vi "试剂余量展示.vi"(11 "波形图 2":refnum<vi>) -> (3 "波形图":sgl[][](graph))   [LabVIEW 2016, in "斯坦道氟化物.lvlib"]
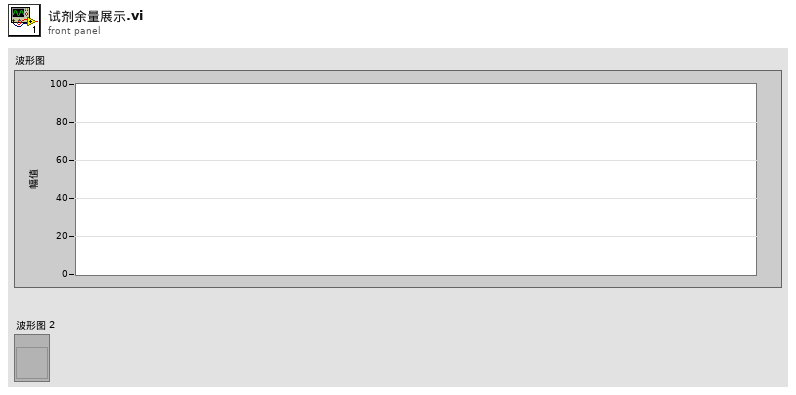
[diagram p1: front panel]
types:
  T1 = cluster{"Name":string, "Color":u32, "Style":u8, "Point Style":u8, "Name Visible":bool, "Allow Drag":bool, "Annotation Mode":u32, "Plot":i32, "Index":i32, "Position":cluster{"X":dbl, "Y":i32}, "X Scale":u32, "Y Scale":u32, "Show Arrow":bool, "Lock Name":bool, "Plot Area":i32, "Label Offset":cluster{"X":dbl, "Y":dbl}}[]
  T2 = cluster{"V1":sgl, "V2":sgl, "V3":sgl, "V4":sgl, "V5":sgl, "V6":sgl, "V7":sgl, "V8":sgl, "V9":sgl, "V10":sgl, "V11":sgl, "V12":sgl, "V9-1":sgl, "V9-2":sgl}
  T3 = cluster{"V":string, "V 2":string, "V 3":string, "V 4":string, "V 5":string, "V 6":string, "V 7":string, "V 8":string, "V 9":string, "V 10":string, "V 11":string, "V 12":string, "V9-1":string, "V9-2":string}
  T4 = cluster{"Name":string, "Color":u32, "Style":u8, "Point Style":u8, "Name Visible":bool, "Allow Drag":bool, "Annotation Mode":u32, "Plot":i32, "Index":i32, "Position":cluster{"X":dbl, "Y":i32}, "X Scale":u32, "Y Scale":u32, "Show Arrow":bool, "Lock Name":bool, "Plot Area":i32, "Label Offset":cluster{"X":dbl, "Y":dbl}}
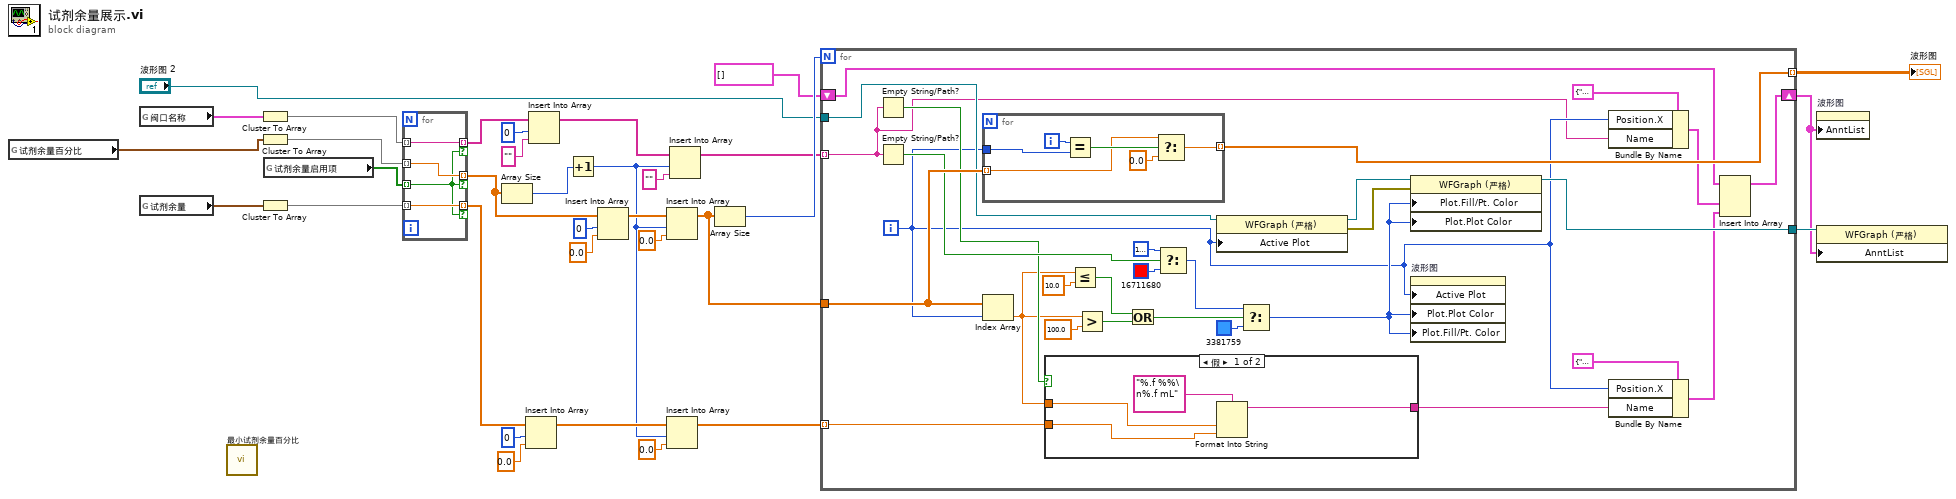
[diagram p0: block diagram]
diagram:
  n1 = global read "VAR总磷总氮全局变量.vi" "试剂余量百分比"() -> (w33:T2)
  n2 = global read "总磷总氮断电保存全局变量.vi" "阀口名称"() -> (w22:T3)
  n3 = global read "VAR总磷总氮全局变量.vi" "试剂余量"() -> (w11:T2)
  n4 = call "最小试剂余量百分比.vi"() -> ()  [unwired: 12 in]
  n5 = Cluster To Array(cluster=w22) -> (array=w21:string[])
  n6 = Cluster To Array(cluster=w33) -> (array=w32:sgl[])
  n7 = Cluster To Array(cluster=w11) -> (array=w10:sgl[])
  n8 = global read "VAR总磷总氮全局变量.vi" "试剂余量启用项"() -> (w31:bool[])
  n9 = for {
    tunnel: w32 -> [w37] mode=indexing
    tunnel: w31 -> [w34] mode=indexing
    tunnel: [w37] -> w30 mode=indexing if=w34
    tunnel: w21 -> [w36] mode=indexing
    tunnel: [w36] -> w20 mode=indexing if=w34
    tunnel: w10 -> [w35] mode=indexing
    tunnel: [w35] -> w5 mode=indexing if=w34
  }
  n10 = Array Size(array=w30) -> (size(s)=w17:i32)
  n11 = Insert Into Array(array=w5, index=0 ("索引"), new element=sgl 0.0 ("新元素/子数组")) -> (w7:sgl[])
  n12 = Insert Into Array(array=w20, index=0 ("索引"), new element="" ("新元素/子数组")) -> (w18:string[])
  n13 = Increment(x=w17) -> (x+1=w4:i32)
  n14 = Insert Into Array(array=w30, index=0 ("索引"), new element=sgl 0.0 ("新元素/子数组")) -> (w28:sgl[])
  n15 = Insert Into Array(array=w28, index=w4, new element=sgl 0.0 ("新元素/子数组")) -> (w24:sgl[])
  n16 = Insert Into Array(array=w7, index=w4, new element=sgl 0.0 ("新元素/子数组")) -> (w3:sgl[])
  n17 = Insert Into Array(array=w18, index=w4, new element="" ("新元素/子数组")) -> (w14:string[])
  n18 = Array Size(array=w24) -> (size(s)=w25:i32)
  n19 = for {
    N: w25 -> [_]
    tunnel: w24 -> [w62]
    tunnel: [w66] -> w23 mode=indexing
    tunnel: w14 -> [w42] mode=indexing
    tunnel: "波形图 2" -> [w55]
    tunnel: [w53] -> w12
    tunnel: w3 -> [w52] mode=indexing
    shift-right: [w38] -> w2
    shift-left: T1 [] -> [w41]
    i -> [w43]
    n20 = Empty String/Path?(string/path=w42) -> (empty?=w50:bool)
    n21 = Empty String/Path?(string/path=w42) -> (empty?=w59:bool)
    n22 = for {
      tunnel: w62 -> [w73] mode=indexing
      tunnel: [w72] -> w66 mode=indexing
      tunnel: w43 -> [w76]
      i -> [w75]
      n23 = Equal?(x=w75, y=w76) -> (x = y?=w74:bool)
      n24 = Select(t=w73, s=w74, f=sgl 0.0) -> (s? t:f=w72:sgl)
    }
    n25 = Index Array(array=w62, index=w43) -> (element=w48:sgl)
    n26 = case shown="假" w50 {
      tunnel: w48 -> [w69 _]
      tunnel: w52 -> [w68 _]
      tunnel: [w67 _] -> w51
      frame False {
        n27 = Format Into String(format string="%.f %%\n%.f mL" ("格式字符串"), w69, w68) -> (resulting string=w67:string)  [unwired: 2 in, 1 out]
      }
      frame True {
      }
    }
    n28 = Less Or Equal?(x=w48, y=sgl 10.0) -> (x <= y?=w60:bool)
    n29 = Greater?(x=w48, y=sgl 100.0) -> (0:w45:bool)
    n30 = Or(x=w60, y=w45) -> (x .or. y?=w46:bool)
    n31 = Select(t=u32 16777216, s=w59, f=u32 16711680) -> (s? t:f=w56:u32)
    n32 = property on="属性节点" class="WFGraph (严格)"(reference=w55, "Active Plot"=w43) -> (reference out=w54:refnum<vi>, error out=w64:errorcluster)  [unwired: 1 in]
    n33 = Select(t=w56, s=w46, f=u32 3381759) -> (s? t:f=w49:u32)
    n34 = property on="属性节点" class="WFGraph (严格)"(reference=w54, error in=w64, "Plot.Fill/Pt. Color"=w49, "Plot.Plot Color"=w49) -> (reference out=w53:refnum<vi>)  [unwired: 1 out]
    n35 = property on="波形图" class="WFGraph (严格)"("Active Plot"=w43, "Plot.Plot Color"=w49, "Plot.Fill/Pt. Color"=w49) -> ()  [unwired: 2 in, 2 out]
    n36 = Bundle By Name(cluster=T4 {"Name"="", "Color"=0, "Style"=0, "Point Style"=0, "Name Visible"=TRUE, "Allow Drag"=FALSE, "Annotation Mode"=0, "Plot"=0, "Index"=0, "Position"={"X"=0.0, "Y"=80}, "X Scale"=0, "Y Scale"=0, "Show Arrow"=FALSE, "Lock Name"=FALSE, "Plot Area"=0, "Label Offset"={"X"=0.0, "Y"=0.0}}, "Position.X"=w43, "Name"=w42) -> (w40:T4)
    n37 = Bundle By Name(cluster=T4 {"Name"="", "Color"=0, "Style"=0, "Point Style"=0, "Name Visible"=TRUE, "Allow Drag"=FALSE, "Annotation Mode"=0, "Plot"=0, "Index"=0, "Position"={"X"=0.0, "Y"=20}, "X Scale"=0, "Y Scale"=0, "Show Arrow"=FALSE, "Lock Name"=FALSE, "Plot Area"=0, "Label Offset"={"X"=0.0, "Y"=0.0}}, "Position.X"=w43, "Name"=w51) -> (w39:T4)
    n38 = Insert Into Array(array=w41, new element #1=w40, new element #2=w39) -> (w38:T1)  [unwired: 1 in]
  }
  "波形图" <- w23
  n39 = property on="波形图" class="WFGraph (严格)"("AnntList"=w2) -> ()  [unwired: 2 in, 2 out]
  n40 = property on="属性节点" class="WFGraph (严格)"(reference=w12, "AnntList"=w2) -> ()  [unwired: 1 in, 2 out]
